vi "CompileMeta.vi"(8 "Compiler Settings":T1={"Python Path"=path "", "Main File"="makesequence.py", "Meta File"="makesequence.py", "Aux File"="makesequence.py"}) -> (0 "Compiler Settings 2":T1={"Python Path"=path "", "Main File"="makesequence.py", "Meta File"="makesequence.py", "Aux File"="makesequence.py"})   [LabVIEW 2017]
uses:
  PulseCompiler/CompilerSettings.ctl
panel:
  out "Array":string[](array[string])
  in  "stop":bool
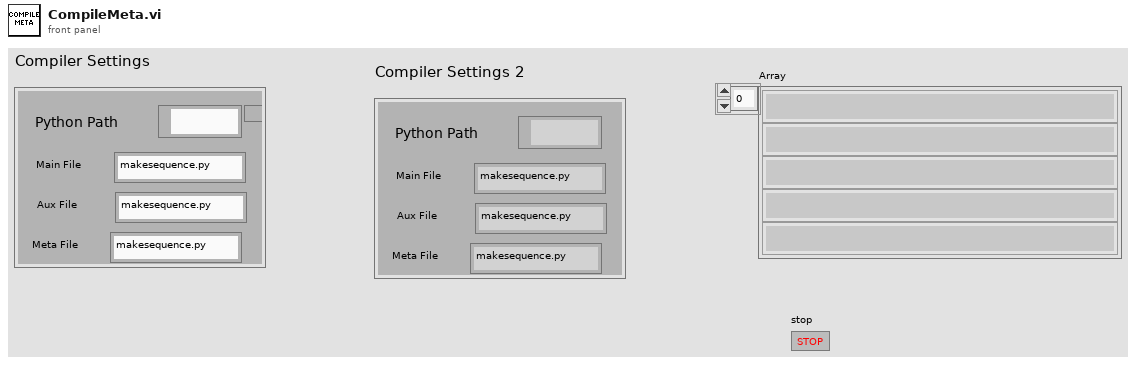
[diagram p1: front panel]
types:
  T1 = typedef "CompilerSettings.ctl" = cluster{"Python Path":path, "Main File":string, "Meta File":string, "Aux File":string}
  T2 = enum16{"open", "replace", "create", "open or create", "replace or create", "replace or create with confirmation"}
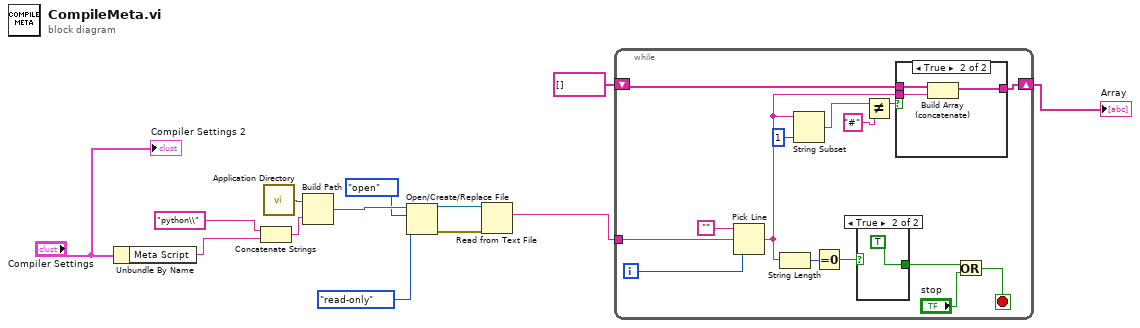
[diagram p0: block diagram]
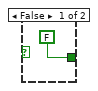
[diagram p3: hidden frame]
diagram:
  n1 = Unbundle By Name("Compiler Settings") -> ("Meta Script"=w9:string)
  n2 = Concatenate Strings("python\\" ("name or relative path"), w9) -> (w11:string)
  n3 = call <vilib>:"Application Directory.vi"() -> ("Application Directory"=w13:path)
  n4 = Build Path(base path=w13, name or relative path=w11) -> (appended path=w12:path)
  n5 = Open/Create/Replace File(file path (use dialog)=w12, operation (0:open)=T2."open", access (0:read/write)=enum16{"read/write", "read-only", "write-only"}."read-only") -> (refnum out=w5:refnum<file>, error out=w6:errorcluster)  [unwired: 3 in, 1 out]
  n6 = Read from Text File(file (use dialog)=w5, error in=w6) -> (text=w3:string)  [unwired: 2 in, 3 out]
  n7 = while {
    shift-right: [w26] -> w2
    shift-left: string[] [] -> [w27]
    tunnel: w3 -> [w19]
    i -> [w28]
    stop <- w20 stop-if-true
    n8 = Pick Line(string ("")="", multi-line string=w19, line index=w28) -> (output string=w15:string)
    n9 = String Length(string=w15) -> (length=w24:i32)
    n10 = String Subset(string=w15, length (rest)=1 ("length (rest)")) -> (substring=w16:string)  [unwired: 1 in]
    n11 = Equal To 0?(x=w24) -> (x = 0?=w23:bool)
    n12 = case shown="True" w23 {
      tunnel: [FALSE TRUE] -> w22
      frame False {
      }
      frame True {
      }
    }
    n13 = Not Equal?(x=w16, y="#") -> (x != y?=w18:bool)
    n14 = case shown="True" w18 {
      tunnel: w27 -> [w29 w32]
      tunnel: [w29 w31] -> w26
      tunnel: w15 -> [_ w30]
      frame False {
      }
      frame True {
        n15 = Build Array (concatenate)(w32, w30) -> (w31:string[])
      }
    }
    n16 = Or(x=w22, y="stop") -> (x .or. y?=w20:bool)
  }
  "Array" <- w2
  "Compiler Settings 2" <- "Compiler Settings"
